vi "initiate.vi"(8 "error in (no error)":errorcluster, 11 "reference in":refnum<class "Master Controller.lvclass">) -> (0 "error out":errorcluster, 3 "reference out":refnum<class "Master Controller.lvclass">)   [LabVIEW 2015, in "Master Controller.lvclass"]
uses:
  Master Controller.lvclass
  File Controller_llb/File Controller.lvclass
  GUI/GUI Controller_llb/GUI Controller.lvclass
  Subject Controller_llb/Subject Controller.lvclass
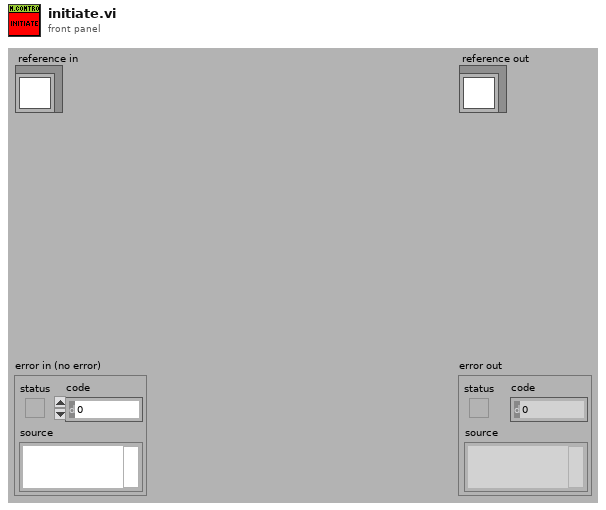
[diagram p1: front panel]
types:
  T1 = typedef "Master Controller.lvclass/ObjectAttributesRef.ctl" = refnum<data-value>
  T2 = typedef "Master Controller.lvclass/ObjectAttributes.ctl" = cluster{"MyAttribute":dbl, "gui_controller_ref":refnum<class "GUI Controller.lvclass">, "file_controller_ref":refnum<class "File Controller.lvclass">, "subject_controller_ref":refnum<class "Subject Controller.lvclass">}
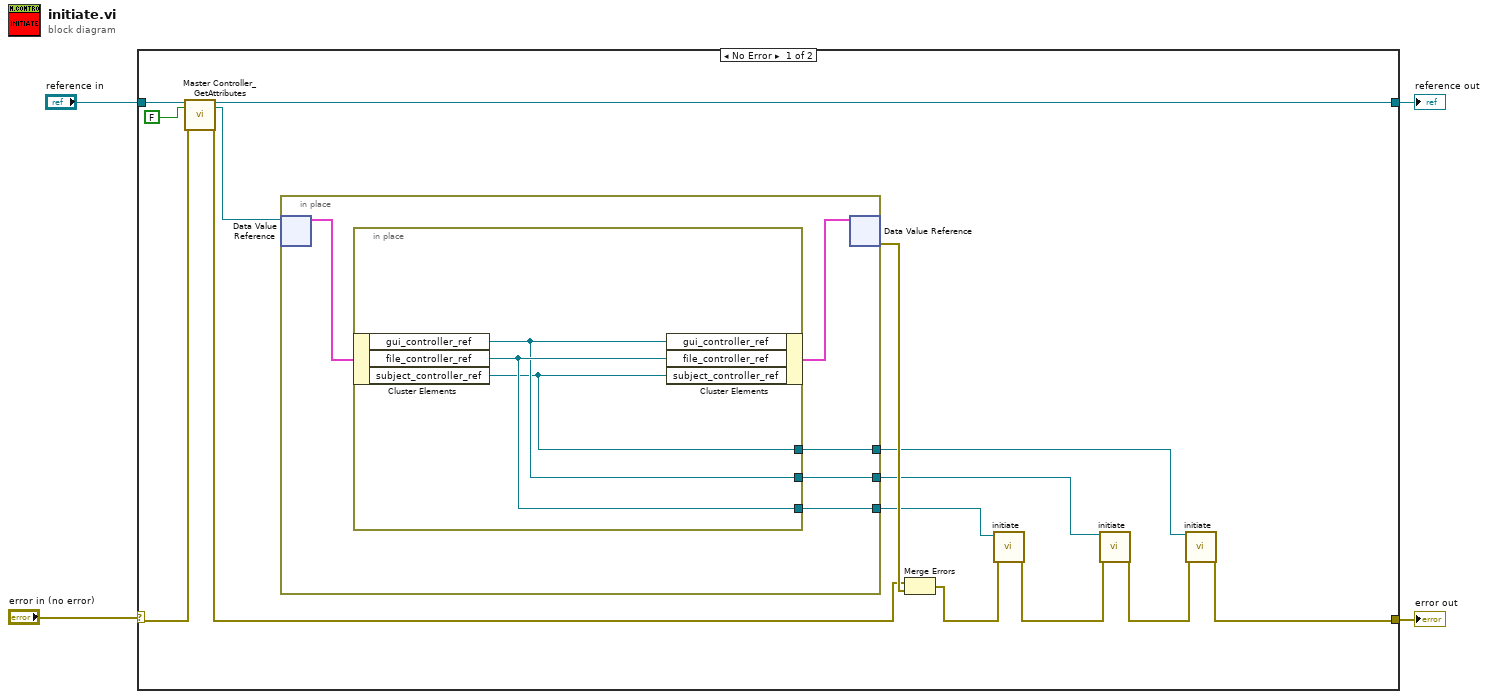
[diagram p0: block diagram]
diagram:
  n1 = case shown="No Error" "error in (no error)" {
    selector: "error in (no error)" -> [w16 w28]
    tunnel: [w5 w28] -> w3
    tunnel: [w15 w27] -> w1
    tunnel: "reference in" -> [w18 w27]
    frame No Error {
      n2 = call "Master Controller_GetAttributes.vi"("reference in"=w18, "return data? (T)"=FALSE, "error in (no error)"=w16) -> ("reference out"=w15:refnum<class "Master Controller.lvclass">, "attributes ref"=w14:T1, "error out"=w12:errorcluster)  [unwired: 13 in, 1 out]
      n3 = in-place {
        in-place-border: [w21] -> w11
        in-place-border: [w20] -> w9
        in-place-border: [w19] -> w7
        n4 = in-place-dvr #1(w14) -> (w22:T2)  [unwired: 1 out]
        n5 = in-place {
          in-place-border: [w26] -> w21
          in-place-border: [w25] -> w20
          in-place-border: [w24] -> w19
          n6 = in-place-cluster #2(w22) -> ("gui_controller_ref"=w25:refnum<class "GUI Controller.lvclass">, "file_controller_ref"=w26:refnum<class "File Controller.lvclass">, "subject_controller_ref"=w24:refnum<class "Subject Controller.lvclass">)
          n7 = in-place-cluster #2("gui_controller_ref"=w25, "file_controller_ref"=w26, "subject_controller_ref"=w24) -> (w23:T2)
        }
        n8 = in-place-dvr #1(w23) -> (w13:errorcluster)  [unwired: 1 out]
      }
      n9 = Merge Errors(w12, w13) -> (w10:errorcluster)
      n10 = call "initiate.vi"("error in (no error)"=w10, "reference in"=w11) -> ("error out"=w8:errorcluster)  [unwired: 8 in, 1 out]
      n11 = call "initiate.vi"("reference in"=w9, "error in (no error)"=w8) -> ("error out"=w6:errorcluster)  [unwired: 16 in, 1 out]
      n12 = call "initiate.vi"("reference in"=w7, "error in (no error)"=w6) -> ("error out"=w5:errorcluster)  [unwired: 16 in, 1 out]
    }
    frame Error {
    }
  }
  "error out" <- w3
  "reference out" <- w1
